vi "LSX Get Stop Accel.vi"(0 "lLSID":i32, 1 "pdAD":dbl, 5 "pdXD":dbl, 7 "pdYD":dbl, 9 "pdZD":dbl, 11 "error in (no error)":errorcluster) -> (3 "pdAD out":dbl, 4 "function return":i32, 6 "pdXD out":dbl, 8 "pdYD out":dbl, 10 "pdZD out":dbl, 15 "error out":errorcluster)   [LabVIEW 2018, in "Tango.lvlib"]
doc: "TANGOAPI int TANGOCALL LSX_GetStopAccel (int lLSID, double *pdXD, double *pdYD, double *pdZD, double *pdAD);"
uses:
  Tango.lvlib
  SubVIs/Tango_DLL.dll
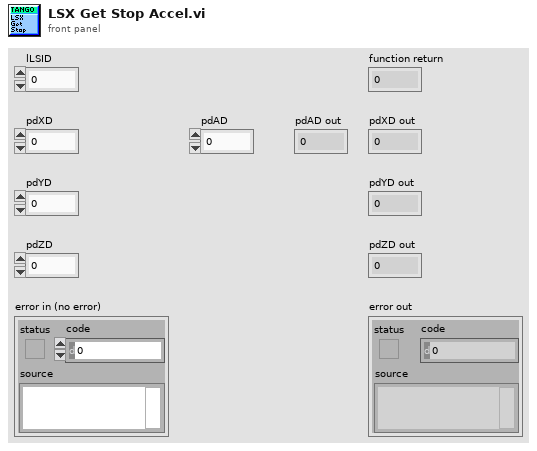
[diagram p1: front panel]
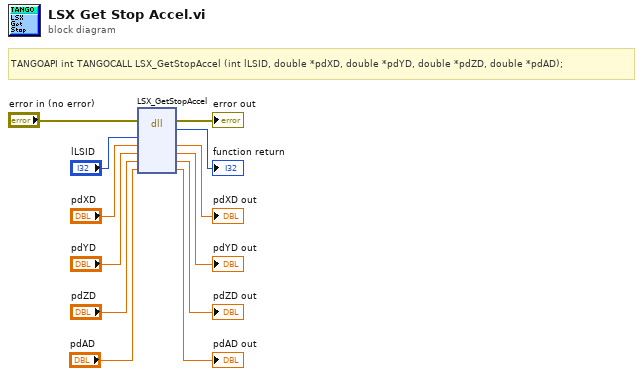
[diagram p0: block diagram]
diagram:
  # "TANGOAPI int TANGOCALL LSX_GetStopAccel (int lLSID, double *pdXD, double *pdYD, double *pdZD, double *pdAD);"
  n1 = dll-call lib="C:/Users/Familie/Documents/LabviewIX81/lib/TANGO Stage/SubVIs/Tango_DLL.*" fn="LSX_GetStopAccel"(error in="error in (no error)", "lLSID"="lLSID", "pdXD"="pdXD", "pdYD"="pdYD", "pdZD"="pdZD", "pdAD"="pdAD") -> (error out=→"error out":errorcluster, →"function return":i32, "pdXD"=→"pdXD out":dbl, "pdYD"=→"pdYD out":dbl, "pdZD"=→"pdZD out":dbl, "pdAD"=→"pdAD out":dbl)  [unwired: 3 in, 1 out]
